vi "Generate Linear Motion Profile.vi"(0 "Initial Snapshot":T5, 1 "Control Boundaries":T3, 2 "Time Between Points (ms)":dbl, 3 "Movement Duration (s)":dbl, 4 "Distance (in)":dbl, 5 "Error In":errorcluster, 6 "Ramp - Velocity and Acceleration Mode":T2, 7 "Ramp - Final Snapshot Request":T1, 8 "Rampup Time (s)":dbl, 9 "Rampdown Time (s)":dbl, 10 "Acceleration (in/s2)":dbl, 11 "Deceleration (in/s2)":dbl, 12 "Cruise Velocity (in/s)":dbl, 13 "Final Velocity (in/s)":dbl) -> (14 "Final Snapshot":T5, 15 "Motion Profile Portion":T4[](array[typedef]), 19 "Error Out":errorcluster)   [LabVIEW 2019, in "Motion Profile Generator.lvclass"]
uses:
  Motion Profile Generator.lvclass
  Type Defs/Motion Snapshot.ctl
  Type Defs/Motion Profile Point.ctl
  Type Defs/Control Boundaries.ctl
  Type Defs/Ramp - Velocity and Acceleration Mode.ctl
  Type Defs/Ramp - Final Snapshot Request.ctl
panel:
  # "To use max velocity and acceleration, then set the velocity and acceleration/deceleration to the max values"
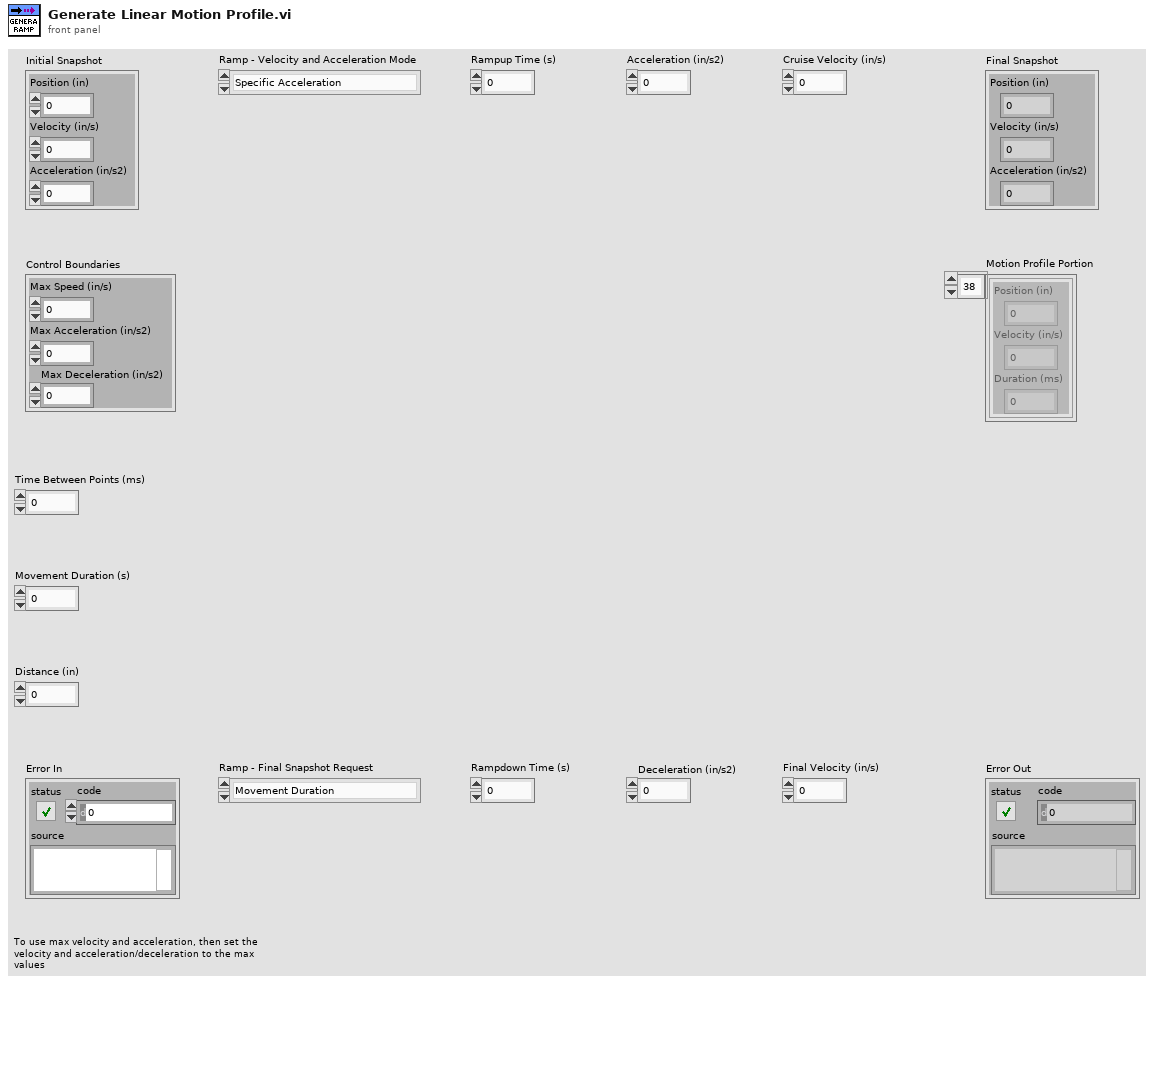
[diagram p1: front panel]
types:
  T1 = typedef "Motion Profile Generator.lvclass/Ramp - Final Snapshot Request.ctl" = enum16{"Movement Duration", "Distance"}
  T2 = typedef "Motion Profile Generator.lvclass/Ramp - Velocity and Acceleration Mode.ctl" = enum16{"Specific Acceleration", "Rampup and Rampdown Times"}
  T3 = typedef "Motion Profile Generator.lvclass/Control Boundaries.ctl" = cluster{"Max Speed (in/s)":dbl, "Max Acceleration (in/s2)":dbl, "Max Deceleration (in/s2)":dbl}
  T4 = typedef "Motion Profile Generator.lvclass/Motion Profile Point.ctl" = cluster{"Position (in)":dbl, "Velocity (in/s)":dbl, "Duration (ms)":dbl}
  T5 = typedef "Motion Profile Generator.lvclass/Motion Snapshot.ctl" = cluster{"Position (in)":dbl, "Velocity (in/s)":dbl, "Acceleration (in/s2)":dbl}
  T6 = cluster{"Ramp - Final Snapshot Request":T1, "Ramp - Velocity and Acceleration Mode":T2, "Distance (in)":dbl, "Movement Duration (s)":dbl, "Initial Snapshot":T5, "Control Boundaries":T3, "Rampup Time (s)":dbl, "Rampdown Time (s)":dbl, "Acceleration (in/s2)":dbl, "Deceleration (in/s2)":dbl, "Cruise Velocity (in/s)":dbl, "Final Velocity (in/s)":dbl, "Time Between Points (ms)":dbl, "Reverse?":bool}
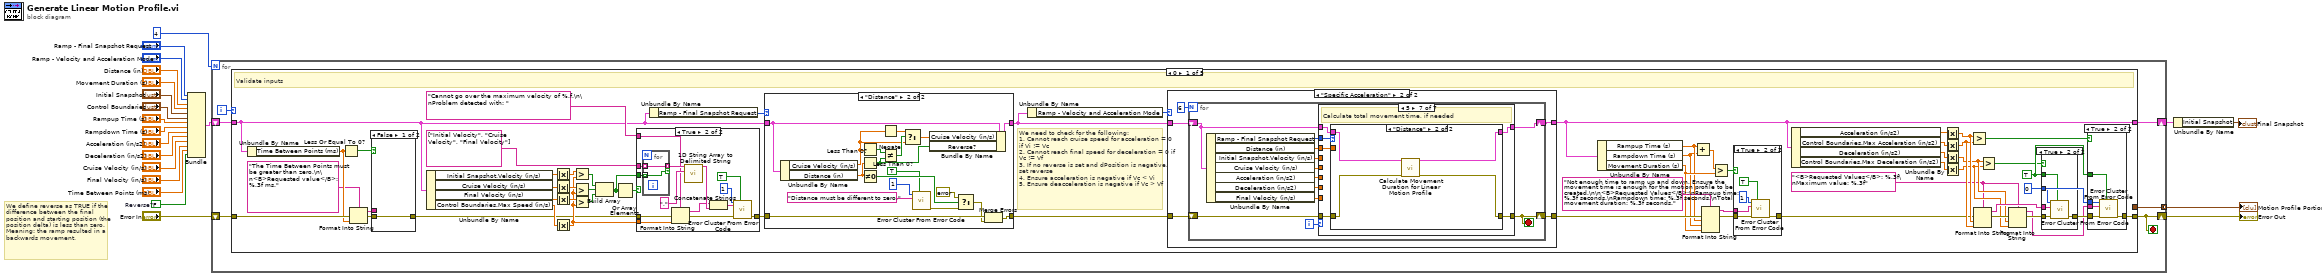
[diagram p0: block diagram]
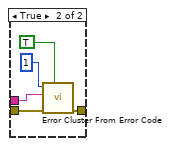
[diagram p2: hidden frame]
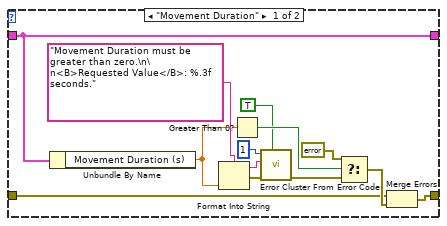
[diagram p4: hidden frame]
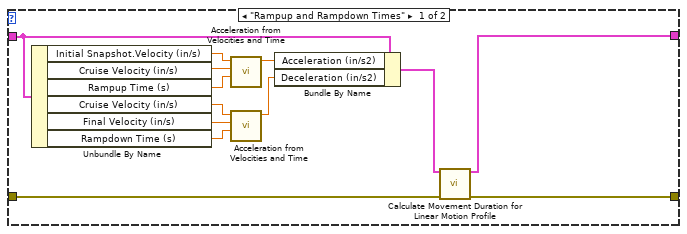
[diagram p5: hidden frame]
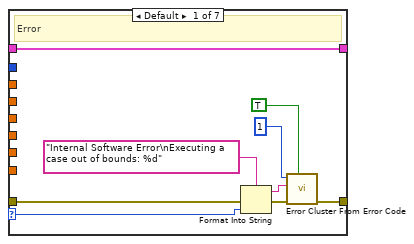
[diagram p6: hidden frame]
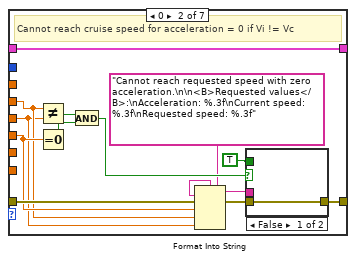
[diagram p7: hidden frame]
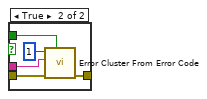
[diagram p8: hidden frame]
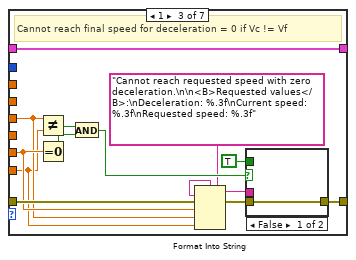
[diagram p9: hidden frame]
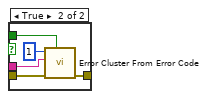
[diagram p10: hidden frame]
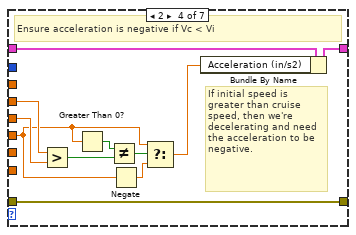
[diagram p11: hidden frame]
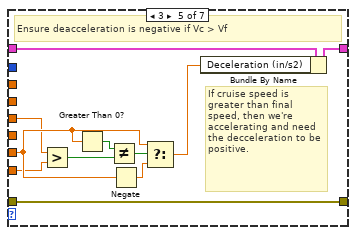
[diagram p12: hidden frame]
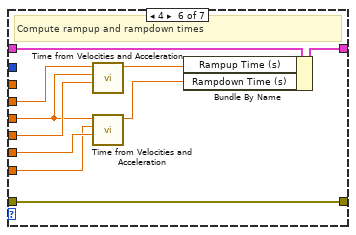
[diagram p13: hidden frame]
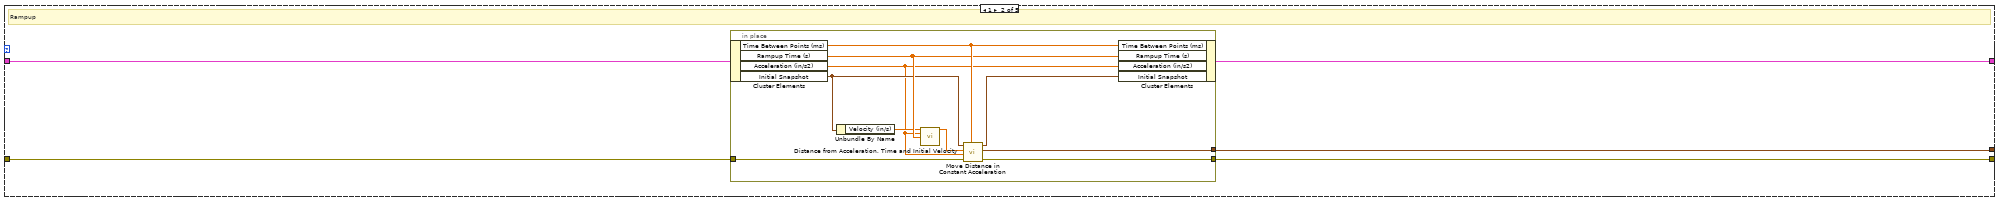
[diagram p18: hidden frame]
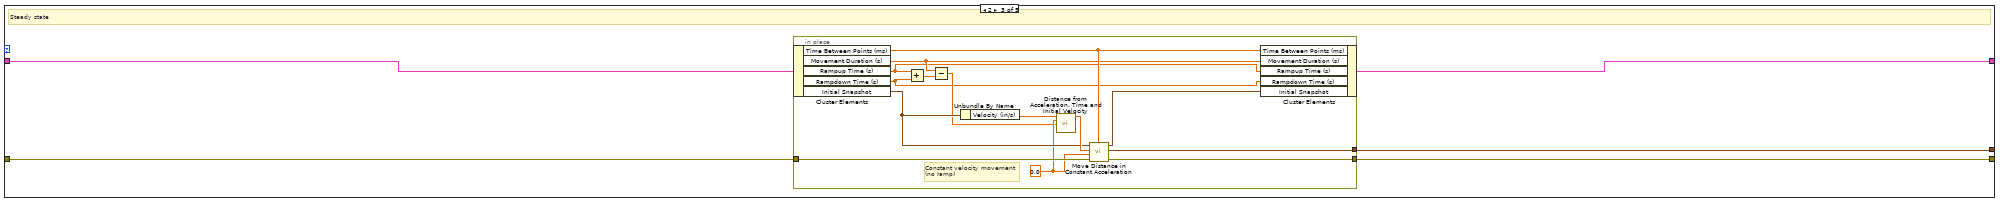
[diagram p19: hidden frame]
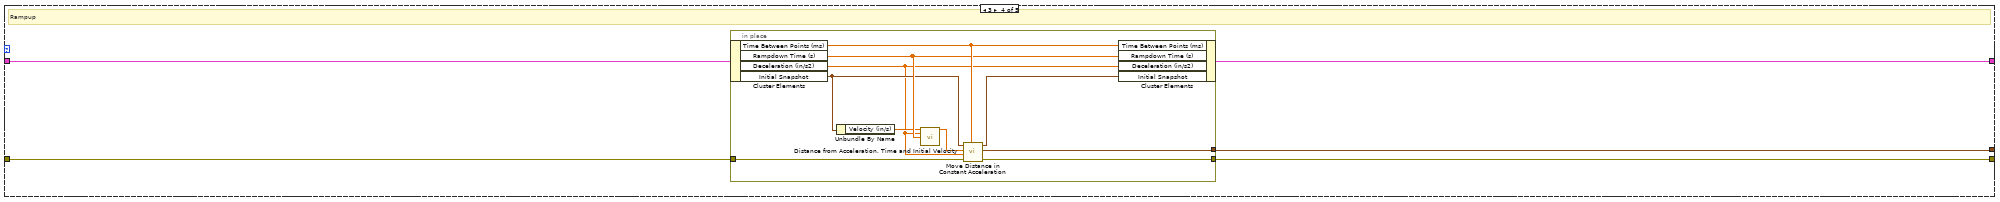
[diagram p20: hidden frame]
diagram:
  w7 = FALSE  # Reverse?
  # "We define reverse as TRUE if the difference between the final position and starting position (the position delta) is less than zero. Meaning: the ramp resulted in a backwards movement."
  n1 = Bundle("Ramp - Final Snapshot Request"="Ramp - Final Snapshot Request", "Ramp - Velocity and Acceleration Mode"="Ramp - Velocity and Acceleration Mode", "Distance (in)"="Distance (in)", "Movement Duration (s)"="Movement Duration (s)", "Initial Snapshot"="Initial Snapshot", "Control Boundaries"="Control Boundaries", "Rampup Time (s)"="Rampup Time (s)", "Rampdown Time (s)"="Rampdown Time (s)", "Acceleration (in/s2)"="Acceleration (in/s2)", "Deceleration (in/s2)"="Deceleration (in/s2)", "Cruise Velocity (in/s)"="Cruise Velocity (in/s)", "Final Velocity (in/s)"="Final Velocity (in/s)", "Time Between Points (ms)"="Time Between Points (ms)", "Reverse?"=w7) -> (w6:T6)  [unwired: 1 in]
  n2 = for {
    N: 4 -> [_]
    shift-right: [w25] -> w20
    shift-left: "Error In" -> [w26]
    shift-right: [w24] -> w2
    shift-left: w6 -> [w23]
    tunnel: [w22] -> w3 mode=concatenating
    i -> [w27]
    stop <- w25 stop-if-true
    n3 = case shown="0" w27 {
      selector: w27 -> [_ _ _ _ w328]
      tunnel: [w58 w280 w295 w314 w334] -> w25
      tunnel: w26 -> [w34 w281 w296 w315 w335]
      tunnel: [w39 w282 w298 w316 w332] -> w24
      tunnel: w23 -> [w35 w283 w297 w317 w332]
      tunnel: [_ w279 w294 w313 _] -> w22
      frame 0 {
        w49 = "<B>Requested Values</B>: %.3f\nMaximum value: %.3f" ("format string")
        w56 = 0 ("error code (0)")
        w57 = TRUE ("show call chain? (False)")
        # "We need to check for the following:\n1. Cannot reach cruise speed for acceleration = 0 if Vi != Vc\n2. Cannot reach final speed for deceleration = 0 if Vc != Vf\n3. If no reverse is set and dPosition is negative, set reverse\n4. Ensure acceleration is negative if Vc < Vi\n5. Ensure deacceleration is negative if Vc > Vf"
        # "Validate inputs"
        n4 = Unbundle By Name(w35) -> ("Time Between Points (ms)"=w30:dbl)
        n5 = Less Or Equal To 0?(x=w30) -> (x <= 0?=w28:bool)
        n6 = Format Into String(format string="The Time Between Points must be greater than zero.\n\n<B>Requested value</B>: %.3f ms.", error in=w34, w30) -> (resulting string=w31:string, error out=w32:errorcluster)  [unwired: 1 in]
        n7 = case shown="False" w28 {
          tunnel: [w86 w89] -> w33
          tunnel: w32 -> [w86 w88]
          tunnel: w31 -> [_ w87]
          frame False {
          }
          frame True {
            n8 = call <vilib>:"Error Cluster From Error Code.vi"("show call chain? (False)"=TRUE, "error in (no error)"=w88, "error message (\"\")"=w87, "error code (0)"=1) -> ("error out"=w89:errorcluster)  [unwired: 5 in]
          }
        }
        n9 = Unbundle By Name(w35) -> ("Initial Snapshot.Velocity (in/s)"=w81:dbl, "Cruise Velocity (in/s)"=w80:dbl, "Final Velocity (in/s)"=w79:dbl, "Control Boundaries.Max Speed (in/s)"=w71:dbl)
        n10 = Absolute Value(x=w81) -> (abs(x)=w69:dbl)
        n11 = Absolute Value(x=w80) -> (abs(x)=w68:dbl)
        n12 = Absolute Value(x=w79) -> (abs(x)=w67:dbl)
        n13 = Absolute Value(x=w71) -> (abs(x)=w62:dbl)
        n14 = Greater?(x=w69, y=w62) -> (0:w78:bool)
        n15 = Greater?(x=w68, y=w62) -> (0:w77:bool)
        n16 = Greater?(x=w67, y=w62) -> (0:w76:bool)
        n17 = Build Array(w78, w77, w76) -> (w72:bool[])
        n18 = Or Array Elements(Boolean array=w72) -> (logical OR=w74:bool)
        n19 = case shown="True" w74 {
          tunnel: w33 -> [w92 w106]
          tunnel: [w92 w105] -> w75
          tunnel: string[] ["Initial Velocity", "Cruise Velocity", "Final Velocity"] -> [_ w104]
          tunnel: w72 -> [_ w103]
          tunnel: w62 -> [_ w94]
          tunnel: "Cannot go over the maximum velocity of %.f.\n\nProblem detected with: " -> [_ w93]
          frame False {
          }
          frame True {
            n20 = for {
              tunnel: w104 -> [w108] mode=indexing
              tunnel: [w108] -> w102 mode=indexing if=w107
              tunnel: w103 -> [w107] mode=indexing
            }
            n21 = Format Into String(format string=w93, error in=w106, w94) -> (resulting string=w95:string, error out=w96:errorcluster)  [unwired: 1 in]
            n22 = call <vilib>:"1D String Array to Delimited String.vi"("delimiter"=",", "string array"=w102) -> ("delimited string"=w97:string)  [unwired: 9 in]
            n23 = Concatenate Strings(w95, w97) -> (w100:string)
            n24 = call <vilib>:"Error Cluster From Error Code.vi"("show call chain? (False)"=TRUE, "error in (no error)"=w96, "error message (\"\")"=w100, "error code (0)"=1) -> ("error out"=w105:errorcluster)  [unwired: 5 in]
          }
        }
        n25 = Unbundle By Name(w35) -> ("Ramp - Final Snapshot Request"=w84:T1)
        n26 = case shown="\"Distance\"" w84 {
          tunnel: [w121 w129] -> w83
          tunnel: w35 -> [w121 w131]
          tunnel: [w115 w137] -> w85
          tunnel: w75 -> [w114 w139]
          frame "Movement Duration" {
            n27 = Unbundle By Name(w121) -> ("Movement Duration (s)"=w111:dbl)
            n28 = Format Into String(format string="Movement Duration must be greater than zero.\n\n<B>Requested Value</B>: %.3f seconds." ("error message (\"\")"), w111) -> (resulting string=w113:string, error out=w110:errorcluster)  [unwired: 2 in]
            n29 = Greater Than 0?(x=w111) -> (x > 0?=w116:bool)
            n30 = call <vilib>:"Error Cluster From Error Code.vi"("show call chain? (False)"=TRUE, "error in (no error)"=w110, "error message (\"\")"=w113, "error code (0)"=1) -> ("error out"=w118:errorcluster)  [unwired: 5 in]
            n31 = Select(t=errorcluster {"status"=FALSE, "code"=0, "source"=""} ("error constant"), s=w116, f=w118) -> (s? t:f=w120:errorcluster)
            n32 = Merge Errors(w114, w120) -> (w115:errorcluster)
          }
          frame "Distance" {
            n33 = Unbundle By Name(w131) -> ("Cruise Velocity (in/s)"=w122:dbl, "Distance (in)"=w130:dbl)
            n34 = Less Than 0?(x=w122) -> (x < 0?=w123:bool)
            n35 = Less Than 0?(x=w130) -> (x < 0?=w125:bool)
            n36 = Not Equal To 0?(x=w130) -> (x != 0?=w138:bool)
            n37 = Negate(x=w122) -> (-x=w126:dbl)
            n38 = Not Equal?(x=w123, y=w125) -> (x != y?=w124:bool)
            n39 = Select(t=w126, s=w124, f=w122) -> (s? t:f=w127:dbl)
            n40 = call <vilib>:"Error Cluster From Error Code.vi"("show call chain? (False)"=TRUE, "error message (\"\")"="Distance must be different to zero." ("error message (\"\")"), "error code (0)"=1) -> ("error out"=w134:errorcluster)  [unwired: 6 in]
            n41 = Bundle By Name(cluster=w131, "Cruise Velocity (in/s)"=w127, "Reverse?"=w125) -> (w129:T6)
            n42 = Select(t=errorcluster {"status"=FALSE, "code"=0, "source"=""} ("error constant"), s=w138, f=w134) -> (s? t:f=w136:errorcluster)
            n43 = Merge Errors(w139, w136) -> (w137:errorcluster)
          }
        }
        n44 = Unbundle By Name(w83) -> ("Ramp - Velocity and Acceleration Mode"=w82:T2)
        n45 = case shown="\"Specific Acceleration\"" w82 {
          tunnel: [w140 w153] -> w39
          tunnel: w83 -> [w152 w157]
          tunnel: [w142 w155] -> w41
          tunnel: w85 -> [w143 w156]
          frame "Rampup and Rampdown Times" {
            n46 = Unbundle By Name(w152) -> ("Initial Snapshot.Velocity (in/s)"=w151:dbl, "Cruise Velocity (in/s)"=w150:dbl, "Rampup Time (s)"=w145:dbl, "Cruise Velocity (in/s)"=w149:dbl, "Final Velocity (in/s)"=w148:dbl, "Rampdown Time (s)"=w144:dbl)
            n47 = call "Acceleration from Velocities and Time.vi"("Time (s)"=w145, "Final Velocity (in/s)"=w150, "Initial Velocity (in/s)"=w151) -> ("Acceleration (in/s2)"=w147:dbl)  [unwired: 8 in]
            n48 = call "Acceleration from Velocities and Time.vi"("Time (s)"=w144, "Final Velocity (in/s)"=w148, "Initial Velocity (in/s)"=w149) -> ("Acceleration (in/s2)"=w146:dbl)  [unwired: 8 in]
            n49 = Bundle By Name(cluster=w152, "Acceleration (in/s2)"=w147, "Deceleration (in/s2)"=w146) -> (w141:T6)
            n50 = call "Calculate Movement Duration for Linear Motion Profile.vi"("Cluster in"=w141, "error in"=w143) -> ("Cluster out"=w140:T6, "error out"=w142:errorcluster)  [unwired: 12 in]
          }
          frame "Specific Acceleration" {
            n51 = for {
              N: 6 -> [_]
              shift-right: [w168] -> w155
              shift-left: w156 -> [w169]
              shift-right: [w158] -> w153
              shift-left: w157 -> [w159]
              i -> [w167]
              stop <- w168 stop-if-true
              n52 = Unbundle By Name(w159) -> ("Ramp - Final Snapshot Request"=w166:T1, "Distance (in)"=w165:dbl, "Initial Snapshot.Velocity (in/s)"=w164:dbl, "Cruise Velocity (in/s)"=w163:dbl, "Acceleration (in/s2)"=w161:dbl, "Deceleration (in/s2)"=w162:dbl, "Final Velocity (in/s)"=w160:dbl)
              n53 = case shown="5" w167 {
                selector: w167 -> [w172 _ _ _ _ _ _]
                tunnel: w169 -> [w173 w191 w210 w227 w238 w247 w250]
                tunnel: [w174 w190 w209 w227 w238 w247 w251] -> w168
                tunnel: w166 -> [_ _ _ _ _ _ w254]
                tunnel: w165 -> [_ _ _ _ _ _ w249]
                tunnel: w164 -> [_ w182 _ w218 _ w241 _]
                tunnel: w163 -> [_ w181 w201 w219 w228 w240 _]
                tunnel: w162 -> [_ _ w202 _ w230 w242 _]
                tunnel: w161 -> [_ w183 _ w217 _ w243 _]
                tunnel: w160 -> [_ _ w200 _ w229 w239 _]
                tunnel: w159 -> [w171 w180 w199 w226 w237 w248 w252]
                tunnel: [w171 w180 w199 w225 w236 w246 w253] -> w158
                frame Default {
                  # "Error"
                  n54 = Format Into String(format string="Internal Software Error\nExecuting a case out of bounds: %d" ("error message (\"\")"), error in=w173, w172) -> (resulting string=w176:string, error out=w177:errorcluster)  [unwired: 1 in]
                  n55 = call <vilib>:"Error Cluster From Error Code.vi"("show call chain? (False)"=TRUE, "error in (no error)"=w177, "error message (\"\")"=w176, "error code (0)"=1) -> ("error out"=w174:errorcluster)  [unwired: 5 in]
                }
                frame 0 {
                  # "Cannot reach cruise speed for acceleration = 0 if Vi != Vc"
                  n56 = Not Equal?(x=w182, y=w181) -> (x != y?=w189:bool)
                  n57 = Equal To 0?(x=w183) -> (x = 0?=w188:bool)
                  n58 = And(x=w189, y=w188) -> (x .and. y?=w187:bool)
                  n59 = Format Into String(format string="Cannot reach requested speed with zero acceleration.\n\n<B>Requested values</B>:\nAcceleration: %.3f\nCurrent speed: %.3f\nRequested speed: %.3f", error in=w191, w183, w182, w181) -> (resulting string=w184:string, error out=w186:errorcluster)  [unwired: 1 in]
                  n60 = case shown="False" w187 {
                    tunnel: w186 -> [w192 w197]
                    tunnel: [w192 w196] -> w190
                    tunnel: w184 -> [_ w194]
                    tunnel: TRUE -> [_ w193]
                    frame False {
                    }
                    frame True {
                      n61 = call <vilib>:"Error Cluster From Error Code.vi"("show call chain? (False)"=w193, "error in (no error)"=w197, "error message (\"\")"=w194, "error code (0)"=1) -> ("error out"=w196:errorcluster)  [unwired: 5 in]
                    }
                  }
                }
                frame 1 {
                  # "Cannot reach final speed for deceleration = 0 if Vc != Vf"
                  n62 = Not Equal?(x=w201, y=w200) -> (x != y?=w208:bool)
                  n63 = Equal To 0?(x=w202) -> (x = 0?=w207:bool)
                  n64 = And(x=w208, y=w207) -> (x .and. y?=w206:bool)
                  n65 = Format Into String(format string="Cannot reach requested speed with zero deceleration.\n\n<B>Requested values</B>:\nDeceleration: %.3f\nCurrent speed: %.3f\nRequested speed: %.3f", error in=w210, w202, w201, w200) -> (resulting string=w203:string, error out=w205:errorcluster)  [unwired: 1 in]
                  n66 = case shown="False" w206 {
                    tunnel: w205 -> [w211 w216]
                    tunnel: [w211 w215] -> w209
                    tunnel: w203 -> [_ w213]
                    tunnel: TRUE -> [_ w212]
                    frame False {
                    }
                    frame True {
                      n67 = call <vilib>:"Error Cluster From Error Code.vi"("show call chain? (False)"=w212, "error in (no error)"=w216, "error message (\"\")"=w213, "error code (0)"=1) -> ("error out"=w215:errorcluster)  [unwired: 5 in]
                    }
                  }
                }
                frame 2 {
                  # "If initial speed is greater than cruise speed, then we're decelerating and need the acceleration to be negative."
                  # "Ensure acceleration is negative if Vc < Vi"
                  n68 = Greater?(x=w218, y=w219) -> (0:w220:bool)
                  n69 = Greater Than 0?(x=w217) -> (x > 0?=w224:bool)
                  n70 = Not Equal?(x=w224, y=w220) -> (x != y?=w223:bool)
                  n71 = Negate(x=w217) -> (-x=w221:dbl)
                  n72 = Select(t=w217, s=w223, f=w221) -> (s? t:f=w222:dbl)
                  n73 = Bundle By Name(cluster=w226, "Acceleration (in/s2)"=w222) -> (w225:T6)
                }
                frame 3 {
                  # "If cruise speed is greater than final speed, then we're accelerating and need the decceleration to be positive."
                  # "Ensure deacceleration is negative if Vc > Vf"
                  n74 = Greater?(x=w228, y=w229) -> (0:w231:bool)
                  n75 = Greater Than 0?(x=w230) -> (x > 0?=w235:bool)
                  n76 = Not Equal?(x=w235, y=w231) -> (x != y?=w234:bool)
                  n77 = Negate(x=w230) -> (-x=w232:dbl)
                  n78 = Select(t=w230, s=w234, f=w232) -> (s? t:f=w233:dbl)
                  n79 = Bundle By Name(cluster=w237, "Deceleration (in/s2)"=w233) -> (w236:T6)
                }
                frame 4 {
                  # "Compute rampup and rampdown times"
                  n80 = call "Time from Velocities and Acceleration.vi"("Acceleration (in/s2)"=w243, "Final Velocity (in/s)"=w240, "Initial Velocity (in/s)"=w241) -> ("Time (s)"=w245:dbl)  [unwired: 8 in]
                  n81 = call "Time from Velocities and Acceleration.vi"("Acceleration (in/s2)"=w242, "Final Velocity (in/s)"=w239, "Initial Velocity (in/s)"=w240) -> ("Time (s)"=w244:dbl)  [unwired: 8 in]
                  n82 = Bundle By Name(cluster=w248, "Rampup Time (s)"=w245, "Rampdown Time (s)"=w244) -> (w246:T6)
                }
                frame 5 {
                  # "Calculate total movement time, if needed"
                  n83 = case shown="\"Distance\"" w254 {
                    tunnel: [w256 w260] -> w253
                    tunnel: w252 -> [w256 w259]
                    tunnel: [w255 w257] -> w251
                    tunnel: w250 -> [w255 w258]
                    tunnel: w249 -> [_ _]
                    frame "Movement Duration" {
                    }
                    frame "Distance" {
                      n84 = call "Calculate Movement Duration for Linear Motion Profile.vi"("Cluster in"=w259, "error in"=w258) -> ("Cluster out"=w260:T6, "error out"=w257:errorcluster)  [unwired: 12 in]
                    }
                  }
                }
              }
            }
          }
        }
        n85 = Unbundle By Name(w39) -> ("Rampup Time (s)"=w37:dbl, "Rampdown Time (s)"=w36:dbl, "Movement Duration (s)"=w38:dbl)
        n86 = Add(x=w37, y=w36) -> (x+y=w46:dbl)
        n87 = Format Into String(format string="Not enough time to ramp up and down. Ensure the movement time is enough for the motion profile to be created.\n\n<B>Requested Values</B>:\nRampup time: %.3f seconds.\nRampdown time: %.3f seconds.\nTotal movement duration: %.3f seconds.", error in=w41, w37, w36, w38) -> (resulting string=w43:string, error out=w44:errorcluster)  [unwired: 1 in]
        n88 = Greater?(x=w46, y=w38) -> (0:w45:bool)
        n89 = case shown="True" w45 {
          tunnel: w44 -> [w261 w266]
          tunnel: [w261 w265] -> w40
          tunnel: w43 -> [_ w262]
          frame False {
          }
          frame True {
            n90 = call <vilib>:"Error Cluster From Error Code.vi"("show call chain? (False)"=TRUE, "error in (no error)"=w266, "error message (\"\")"=w262, "error code (0)"=1) -> ("error out"=w265:errorcluster)  [unwired: 5 in]
          }
        }
        n91 = Unbundle By Name(w39) -> ("Acceleration (in/s2)"=w66:dbl, "Control Boundaries.Max Acceleration (in/s2)"=w65:dbl, "Deceleration (in/s2)"=w64:dbl, "Control Boundaries.Max Deceleration (in/s2)"=w63:dbl)
        n92 = Absolute Value(x=w66) -> (abs(x)=w53:dbl)
        n93 = Absolute Value(x=w65) -> (abs(x)=w52:dbl)
        n94 = Absolute Value(x=w64) -> (abs(x)=w51:dbl)
        n95 = Absolute Value(x=w63) -> (abs(x)=w50:dbl)
        n96 = Greater?(x=w53, y=w52) -> (0:w47:bool)
        n97 = Format Into String(format string=w49, error in=w40, w53, w52) -> (resulting string=w55:string, error out=w61:errorcluster)  [unwired: 1 in]
        n98 = Greater?(x=w51, y=w50) -> (0:w48:bool)
        n99 = Format Into String(format string=w49, error in=w61, w51, w50) -> (resulting string=w54:string, error out=w60:errorcluster)  [unwired: 1 in]
        n100 = case shown="True" w48 {
          tunnel: w60 -> [w273 w278]
          tunnel: [w273 w277] -> w59
          tunnel: w57 -> [_ w276]
          tunnel: w56 -> [_ w275]
          tunnel: w55 -> [_ w274]
          frame False {
          }
          frame True {
            n101 = call <vilib>:"Error Cluster From Error Code.vi"("show call chain? (False)"=w276, "error in (no error)"=w278, "error message (\"\")"=w274, "error code (0)"=w275) -> ("error out"=w277:errorcluster)  [unwired: 5 in]
          }
        }
        n102 = case shown="True" w47 {
          tunnel: w59 -> [w267 w272]
          tunnel: [w267 w271] -> w58
          tunnel: w57 -> [_ w270]
          tunnel: w56 -> [_ w269]
          tunnel: w54 -> [_ w268]
          frame False {
          }
          frame True {
            n103 = call <vilib>:"Error Cluster From Error Code.vi"("show call chain? (False)"=w270, "error in (no error)"=w272, "error message (\"\")"=w268, "error code (0)"=w269) -> ("error out"=w271:errorcluster)  [unwired: 5 in]
          }
        }
      }
      frame 1 {
        # "Rampup"
        n104 = in-place {
          in-place-border: [w292] -> w280
          in-place-border: w281 -> [w293]
          in-place-border: [w289] -> w279
          n105 = in-place-cluster #1(w283) -> ("Time Between Points (ms)"=w290:dbl, "Rampup Time (s)"=w287:dbl, "Acceleration (in/s2)"=w284:dbl, "Initial Snapshot"=w286:T5)
          n106 = Unbundle By Name(w286) -> ("Velocity (in/s)"=w285:dbl)
          n107 = call "Distance from Acceleration, Time and Initial Velocity.vi"("Initial Velocity (in/s)"=w285, "Acceleration (in/s2)"=w284, "Time (s)"=w287) -> ("Distance (in)"=w288:dbl)  [unwired: 12 in]
          n108 = call "Move Distance in Constant Acceleration.vi"("Time Between Points (ms)"=w290, "Error In"=w293, "Acceleration (in/s2)"=w284, "Distance (in)"=w288, "Initial Snapshot"=w286) -> ("Error Out"=w292:errorcluster, "Motion Profile Portion"=w289:T4[], "Final Snapshot"=w291:T5)  [unwired: 3 in, 1 out]
          n109 = in-place-cluster #1("Time Between Points (ms)"=w290, "Rampup Time (s)"=w287, "Acceleration (in/s2)"=w284, "Initial Snapshot"=w291) -> (w282:T6)
        }
      }
      frame 2 {
        # "Steady state"
        n110 = in-place {
          in-place-border: [w311] -> w295
          in-place-border: w296 -> [w312]
          in-place-border: [w299] -> w294
          w305 = 0.0 ("Acceleration (in/s2)")
          # "Constant velocity movement\n(no ramp)"
          n111 = in-place-cluster #2(w297) -> ("Time Between Points (ms)"=w310:dbl, "Movement Duration (s)"=w302:dbl, "Rampup Time (s)"=w301:dbl, "Rampdown Time (s)"=w300:dbl, "Initial Snapshot"=w306:T5)
          n112 = Add(x=w301, y=w300) -> (x+y=w309:dbl)
          n113 = Subtract(x=w302, y=w309) -> (x-y=w303:dbl)
          n114 = Unbundle By Name(w306) -> ("Velocity (in/s)"=w304:dbl)
          n115 = call "Distance from Acceleration, Time and Initial Velocity.vi"("Initial Velocity (in/s)"=w304, "Acceleration (in/s2)"=w305, "Time (s)"=w303) -> ("Distance (in)"=w308:dbl)  [unwired: 12 in]
          n116 = call "Move Distance in Constant Acceleration.vi"("Time Between Points (ms)"=w310, "Error In"=w312, "Acceleration (in/s2)"=w305, "Distance (in)"=w308, "Initial Snapshot"=w306) -> ("Error Out"=w311:errorcluster, "Motion Profile Portion"=w299:T4[], "Final Snapshot"=w307:T5)  [unwired: 3 in, 1 out]
          n117 = in-place-cluster #2("Time Between Points (ms)"=w310, "Movement Duration (s)"=w302, "Rampup Time (s)"=w301, "Rampdown Time (s)"=w300, "Initial Snapshot"=w307) -> (w298:T6)
        }
      }
      frame 3 {
        # "Rampup"
        n118 = in-place {
          in-place-border: [w326] -> w314
          in-place-border: w315 -> [w327]
          in-place-border: [w323] -> w313
          n119 = in-place-cluster #3(w317) -> ("Time Between Points (ms)"=w324:dbl, "Rampdown Time (s)"=w321:dbl, "Deceleration (in/s2)"=w318:dbl, "Initial Snapshot"=w320:T5)
          n120 = Unbundle By Name(w320) -> ("Velocity (in/s)"=w319:dbl)
          n121 = call "Distance from Acceleration, Time and Initial Velocity.vi"("Initial Velocity (in/s)"=w319, "Acceleration (in/s2)"=w318, "Time (s)"=w321) -> ("Distance (in)"=w322:dbl)  [unwired: 12 in]
          n122 = call "Move Distance in Constant Acceleration.vi"("Time Between Points (ms)"=w324, "Error In"=w327, "Acceleration (in/s2)"=w318, "Distance (in)"=w322, "Initial Snapshot"=w320) -> ("Error Out"=w326:errorcluster, "Motion Profile Portion"=w323:T4[], "Final Snapshot"=w325:T5)  [unwired: 3 in, 1 out]
          n123 = in-place-cluster #3("Time Between Points (ms)"=w324, "Rampdown Time (s)"=w321, "Deceleration (in/s2)"=w318, "Initial Snapshot"=w325) -> (w316:T6)
        }
      }
      frame Default {
        # "Error"
        n124 = Format Into String(format string="Internal Software Error\nExecuting a case out of bounds: %d" ("error message (\"\")"), error in=w335, w328) -> (resulting string=w330:string, error out=w331:errorcluster)  [unwired: 1 in]
        n125 = call <vilib>:"Error Cluster From Error Code.vi"("error in (no error)"=w331, "error message (\"\")"=w330, "error code (0)"=1) -> ("error out"=w334:errorcluster)  [unwired: 6 in]
      }
    }
  }
  "Motion Profile Portion" <- w3
  "Error Out" <- w20
  n126 = Unbundle By Name(w2) -> ("Initial Snapshot"=→"Final Snapshot":T5)
